vi "PicoScope3000aExampleRapidBlockBulkOverlapped.vi"() -> ()   [LabVIEW 2010]
uses:
  shared/PicoBuffers.ctl
  <vilib>/Waveform/DWDTOps.llb/DWDT Analog to Digital.vi
  shared/Segment Range.ctl
  shared/Buffer and Transfer Settings.ctl
  shared/Acquisition Settings.ctl
  shared/nSegments.ctl
  PicoScope3000aLib/PicoScope3000aDigitalChannelSettings.ctl
  PicoScope3000aLib/PicoScope3000aAnalogChannelSettings.ctl
panel:
  in  "timeIntervalRequested":dbl min=0.0 format="%#6_6p"
  in  "roundFaster":bool=TRUE
  in  "Write to TDMS":bool
  in  "Trigger Settings":T1={"Trigger Enabled"=FALSE, "Trigger Source"=enum."Channel A", "Trigger Threshold (volts)"=0.0, "Trigger Direction"=2, "Trigger Delay (samples)"=0, "Auto Trigger Time (ms)"=1000} {"Trigger Direction" items=["Above", "Below", "Rising", "Falling", "Rising or Falling"]}
  in  "Channel A Settings":T2={"Enabled"=TRUE, "Coupling"=1, "Range"=6, "Analogue Offset"=0.0, "Bandwidth Limit"=0} {"Bandwidth Limit" items=["Full", "20MHz"]; "Range" items=["10 mV", "20 mV", "50 mV", "100 mV", "200 mV", "500 mV", "1 V", "2 V", "5 V", "10 V", "20 V", "50 V ", "100 V"]; "Coupling" items=["AC", "DC"]}
  out "overflow":i16[](array[numeric]) format="%06b"
  in  "Port 0 Settings":T3={"Enabled"=FALSE, "Logic Level"=9830} {"Logic Level" items=["1.5V TTL"=9830, "2.5V CMOS"=16383]}
  out "USB 3.0 device on non-USB 3.0 Port":bool=TRUE
  out "USB Powered":bool=TRUE
  out "Device Info":T4={"Driver Version"="2.1.104.3324", "USB Version"="2.0", "Hardware"="1", "Variant"="5244A", "Batch and Serial"="CQ178/007", "Cal Date"="11Jun13", "Kernel Version"="1.0", "Digital HW Version"="1", "Analogue HW Version"="1", "MSO"=FALSE, "Number of channels"=2}
  in  "Stop Display":bool
  out "Capture Complete":bool
  in  "Run":bool
  in  "Display Buffer Index":i32
  in  "Segment Range":T5={"fromSegmentIndex"=0, "toSegmentIndex"=9} {"toSegmentIndex" format="%.4p"; "fromSegmentIndex" format="%.4p"}
  in  "nSegments":T6=10 format="%.4p"
  out "error out":errorcluster
  in  "Data file":path=path "PicoScope3000aExampleRapidBlock Data"
  in  "Buffer and Transfer Settings":T7={"startIndex"=0, "Samples"=1000000, "Down Sample Ratio"=1, "Down-Sample Mode"=0} {"Down-Sample Mode" items=["RAW none"=2147483648, "None"=0, "Aggregate"=1, "Decimate"=2, "Average"=4]; "Down Sample Ratio" step=1; "Samples" format="%_6p"}
  in  "Acquisition Settings":T8={"preTriggerSamples"=0, "postTriggerSamples"=1000000, "timebase"=5} {"postTriggerSamples" format="%_6p"; "preTriggerSamples" format="%_6p"}
  out "Properties Panel":T9={"Sample Frequency"=41666668.0, "Sample Rate"=2.4000000209412065e-08, "Max Samples Available"=26843008, "Number of Samples"=0, "Total Capture Time (sec) "=0.0, "Max Total Capture Time Available (sec)"=0.6442322134971619} {"Max Total Capture Time Available (sec)" format="%.3p"; "Sample Frequency" format="%.6p"; "Sample Rate" format="%.3p"; "Max Samples Available" format="%_6p"; "Total Capture Time (sec)" format="%.3p"}
  out "Port 0":digitalwaveform(graph)={"t0"=timestamp(0 s since 1904-01-01), "dt"=8e-09, "Y"={"transitions"=[], "data"=[]}}
  in  "stop":bool
  out "Analog Channels":cluster{i32, sgl, "Data":dbl[]}[](graph)
  in  "Serial Number":string
  in  "Use Serial Number":bool
  in  "error in (no error)":errorcluster
  # "Number of\nSegments to Capture"
  # "Bit 0 = ChA"
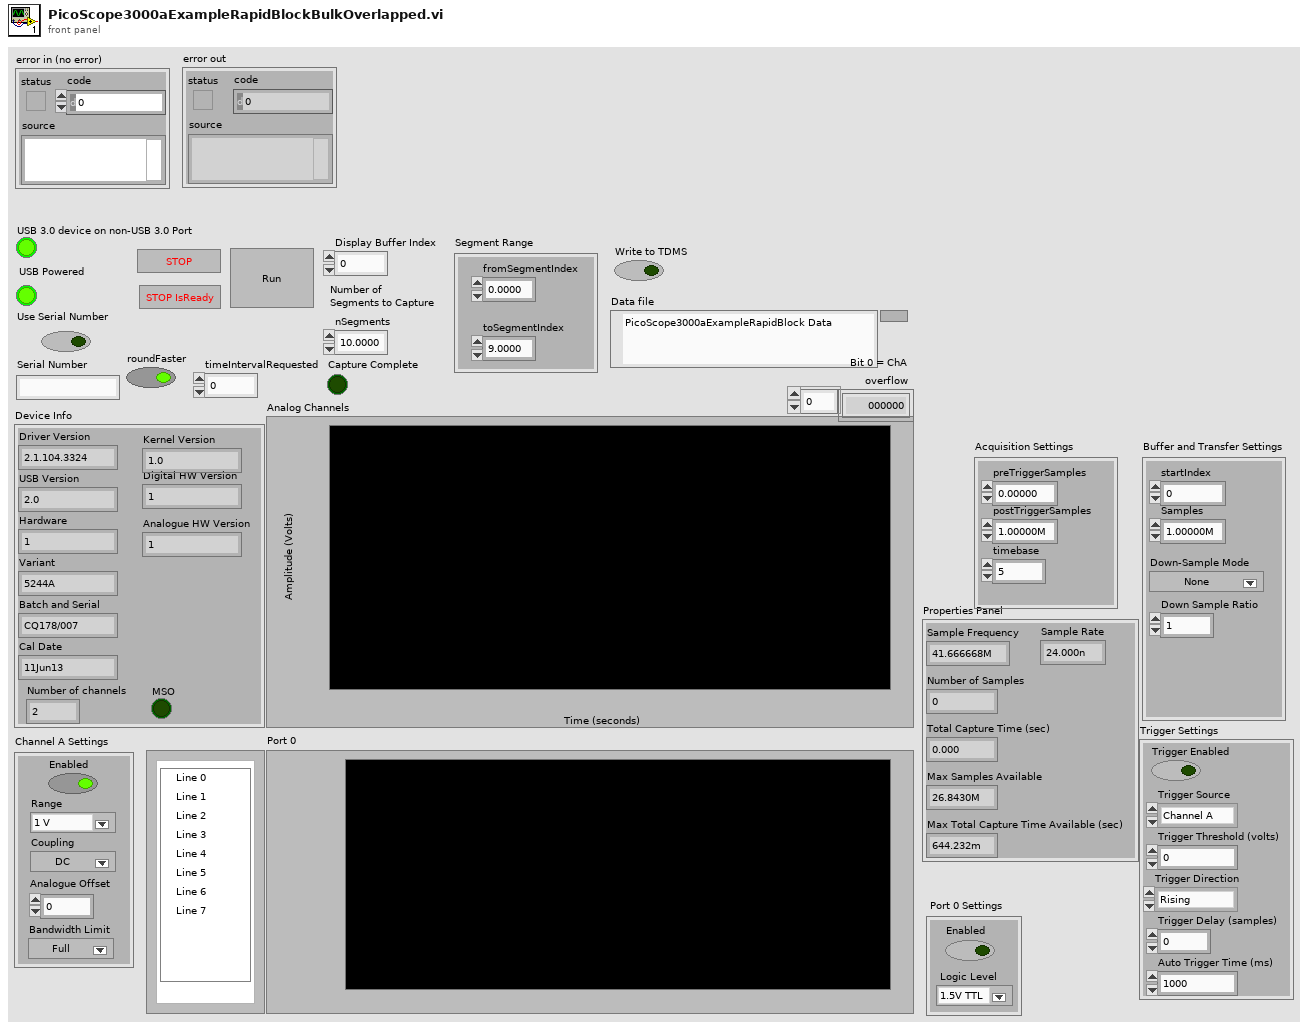
[diagram p1: front panel]
types:
  T1 = cluster{"Trigger Enabled":bool, "Trigger Source":enum32{"Channel A", "Channel B", "Channel C", "Channel D", "Ext."}, "Trigger Threshold (volts)":dbl, "Trigger Direction":u32, "Trigger Delay (samples)":u32, "Auto Trigger Time (ms)":i16}
  T2 = typedef "PicoScope3000aAnalogChannelSettings.ctl" = cluster{"Enabled":bool, "Coupling":u32, "Range":u32, "Analogue Offset":sgl, "Bandwidth Limit":u32}
  T3 = typedef "PicoScope3000aDigitalChannelSettings.ctl" = cluster{"Enabled":bool, "Logic Level":i16}
  T4 = cluster{"Driver Version":string, "USB Version":string, "Hardware":string, "Variant":string, "Batch and Serial":string, "Cal Date":string, "Kernel Version":string, "Digital HW Version":string, "Analogue HW Version":string, "MSO":bool, "Number of channels":i16}
  T5 = typedef "Segment Range.ctl" = cluster{"fromSegmentIndex":u64, "toSegmentIndex":u64}
  T6 = typedef "nSegments.ctl" = u64
  T7 = typedef "Buffer and Transfer Settings.ctl" = cluster{"startIndex":u64, "Samples":u64, "Down Sample Ratio":u64, "Down-Sample Mode":u32}
  T8 = typedef "Acquisition Settings.ctl" = cluster{"preTriggerSamples":u64, "postTriggerSamples":u64, "timebase":u32}
  T9 = cluster{"Sample Frequency":dbl, "Sample Rate":dbl, "Max Samples Available":u64, "Number of Samples":u64, "Total Capture Time (sec) ":dbl, "Max Total Capture Time Available (sec)":dbl}
  T10 = typedef "PicoBuffers.ctl" = cluster{"Max Buffer Pointers":u64[][][], "Min Buffer Pointers":u64[][][], "StreamingDataInfo":cluster{"Channel":u32, "Down-Sample Mode":u32, "PICO_DATA_TYPE":enum32{"PICO_INT8_T", "PICO_INT16_T", "PICO_INT32_T", "PICO_UINT32_T", "PICO_INT64_T", ""}, "Samples":i32, "bufferIndex":u64, "startIndex":i32, "overflow":i16}[][]}
  T11 = enum16{"open", "open or create", "create or replace", "create", "open (read-only)"}
  T12 = cluster{"Sample Frequency":sgl, "Sample Rate":sgl, "Max Samples Available":i32, "Number of Samples":u32, "Total Capture Time (sec) ":sgl, "Max Total Capture Time Available (sec)":sgl}
  T13 = cluster{"Channel A Buffer":i16[], "Channel B Buffer":i16[], "Channel C Buffer":i16[], "Channel D Buffer":i16[], "Channel E Buffer":i16[], "Channel F Buffer":i16[], "Channel G Buffer":i16[], "Channel H Buffer":i16[], "Port 0 Buffer":i16[], "Port 1 Buffer":i16[]}[]
  T14 = cluster{"Channel A Buffer":i16[], "Channel B Buffer":i16[], "Channel C Buffer":i16[], "Channel D Buffer":i16[], "Channel E Buffer":i16[], "Channel F Buffer":i16[], "Channel G Buffer":i16[], "Channel H Buffer":i16[], "Port 0 Buffer":i16[], "Port 1 Buffer":i16[]}
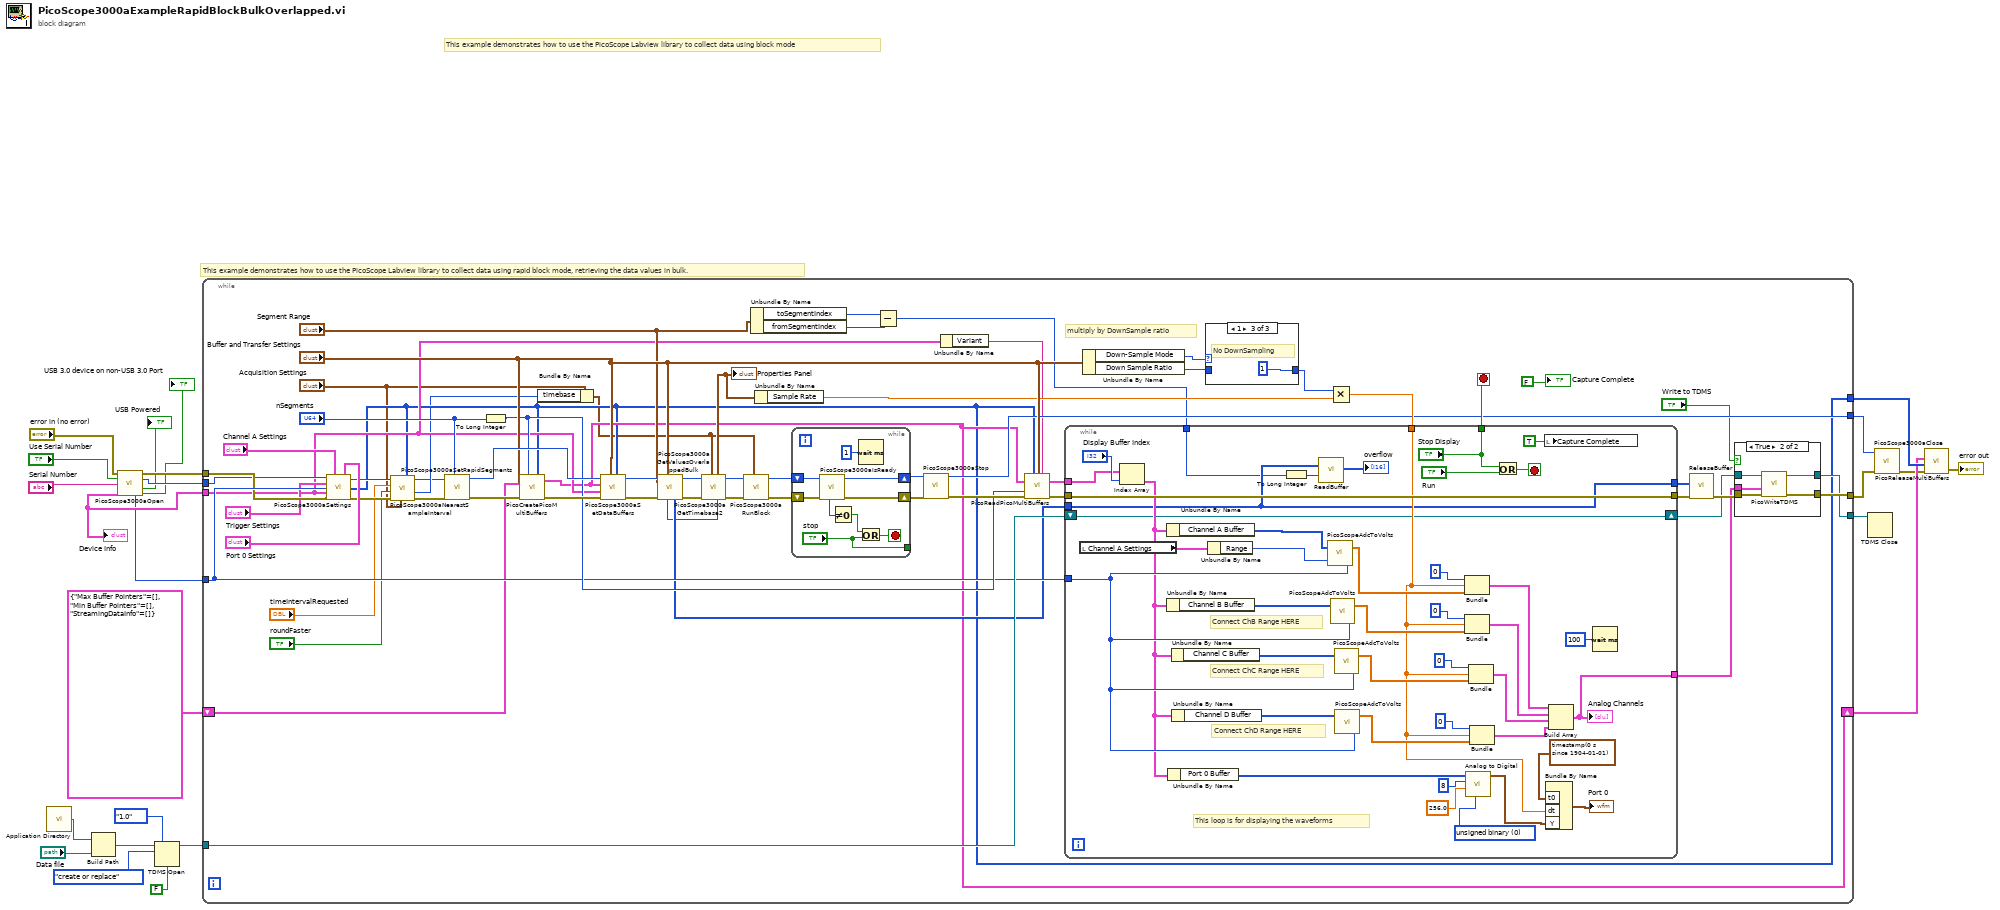
[diagram p0: block diagram]
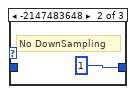
[diagram p4: hidden frame]
diagram:
  # "This example demonstrates how to use the PicoScope Labview library to collect data using rapid block mode, retrieving the data values in bulk."
  # "This example demonstrates how to use the PicoScope Labview library to collect data using block mode"
  n1 = call <vilib>:"Application Directory.vi"() -> ("Application Directory"=w16:path)
  n2 = Build Path(base path=w16, name or relative path="Data file") -> (appended path=w17:path)
  n3 = call "PicoScope3000aOpen.vi"("error in (no error)"="error in (no error)", "Serial Number"="Serial Number", "Use Serial number"="Use Serial Number") -> ("error out"=w8:errorcluster, "handle"=w24:i16, "USB Powered"=→"USB Powered":bool, "Device Info"=w9:T4, "Max ADC value"=w7:i16, "USB 3.0 device on non-USB 3.0 Port"=→"USB 3.0 device on non-USB 3.0 Port":bool)  [unwired: 6 in, 1 out]
  "Device Info" <- w9
  n4 = TDMS Open(6:FALSE ("disable buffering? (T)"), 7:enum16{"1.0", "2.0"}."1.0" ("file format version (2.0)"), 10:T11."create or replace" ("operation (0:open)"), 11:w17) -> (3:w14:refnum<k34>)  [unwired: 2 in, 1 out]
  n5 = while {
    tunnel: w24 -> [w53]
    tunnel: w7 -> [w61]
    tunnel: [w66] -> w22
    tunnel: [w30] -> w23
    tunnel: [w37] -> w15
    tunnel: w14 -> [w86]
    tunnel: w9 -> [w44]
    tunnel: w8 -> [w54]
    tunnel: [w38] -> w2
    shift-right: [w42] -> w3
    shift-left: T10 {"Max Buffer Pointers"=[], "Min Buffer Pointers"=[], "StreamingDataInfo"=[]} ("Data Pointers") -> [w43]
    stop <- w71 stop-if-true
    # "multiply by DownSample ratio"
    n6 = call "PicoScope3000aSettings.vi"("handle in"=w53, "Channel A Settings"="Channel A Settings", "Port 0 Settings"="Port 0 Settings", "Trigger Settings"="Trigger Settings", "Max_adc"=w61, "Device Info"=w44, "error in"=w54) -> ("handle out"=w31:i16, "Enabled Array"=w30:i16[], "error out"=w35:errorcluster)  [unwired: 6 in]
    n7 = call "PicoScope3000aNearestSampleInterval.vi"("Enabled array"=w30, "Acquisition Settings"="Acquisition Settings", "error in (no error)"=w35, "roundFaster"="roundFaster", "timeIntervalRequested"="timeIntervalRequested", "handle in"=w31) -> ("error out"=w34:errorcluster, "timebase"=w27:u32, "handle out"=w26:i16)  [unwired: 2 in, 1 out]
    n8 = call "PicoScope3000aSetRapidSegments.vi"("nSegments"="nSegments", "error in (no error)"=w34, "handle in"=w26) -> ("error out"=w85:errorcluster, "handle out"=w84:i16)  [unwired: 6 in, 1 out]
    n9 = To Long Integer(number="nSegments") -> (32bit integer=w64:i32)
    n10 = call "PicoCreatePicoMultiBuffers.vi"("Number of Buffers"=w64, "Buffer and Transfer Settings"="Buffer and Transfer Settings", "enabled array"=w30, "Data Pointers In"=w43, "error in (no error)"=w85) -> ("Data Pointers"=w42:T10, "error out"=w87:errorcluster)  [unwired: 9 in]
    n11 = Bundle By Name(cluster="Acquisition Settings", "timebase"=w27) -> (w29:T8)
    n12 = call "PicoScope3000aSetDataBuffers.vi"("enabled array"=w30, "Buffer and Transfer Settings"="Buffer and Transfer Settings", "error in (no error)"=w87, "Device Info"=w44, "Data Pointers In"=w42, "handle in"=w84) -> ("error out"=w83:errorcluster, "handle out"=w82:i16)  [unwired: 4 in]
    n13 = call "PicoScope3000aGetValuesOverlappedBulk.vi"("Segment Range"="Segment Range", "Buffer and Transfer Settings"="Buffer and Transfer Settings", "error in (no error)"=w83, "handle in"=w82) -> ("error out"=w58:errorcluster, "handle out"=w57:i16, "Pointer to Overflow"=w50:u64[], "noOfSamples"=w25:u64)  [unwired: 4 in]
    n14 = call "PicoScope3000aGetTimebase2.vi"("Number of Samples"=w25, "Acquisition Settings"=w29, "error in (no error)"=w58, "handle in"=w57) -> ("error out"=w55:errorcluster, "handle out"=w56:i16, "Properties Panel"=w77:T12)  [unwired: 5 in]
    "Properties Panel" <- w77
    n15 = call "PicoScope3000aRunBlock.vi"("Acquisition Settings"=w29, "error in (no error)"=w55, "handle in"=w56) -> ("error out"=w74:errorcluster, "handle out"=w73:i16)  [unwired: 5 in, 2 out]
    n16 = Unbundle By Name("Segment Range") -> ("toSegmentIndex"=w48:u64, "fromSegmentIndex"=w47:u64)
    n17 = Unbundle By Name(w77) -> ("Sample Rate"=w63:sgl)
    n18 = while {
      shift-right: [w144] -> w68
      shift-left: w74 -> [w145]
      shift-right: [w143] -> w65
      shift-left: w73 -> [w142]
      tunnel: ["stop"] -> _
      stop <- w139 stop-if-true
      n19 = call "PicoScope3000aIsReady.vi"("error in (no error)"=w145, "handle in"=w142) -> ("error out"=w144:errorcluster, "handle out"=w143:i16, "ready"=w141:i16)  [unwired: 7 in]
      n20 = Not Equal To 0?(x=w141) -> (x != 0?=w140:bool)
      n21 = Wait (ms)(milliseconds to wait=u32 1) -> ()  [unwired: 1 out]
      n22 = Or(x=w140, y="stop") -> (x .or. y?=w139:bool)
    }
    n23 = Subtract(x=w48, y=w47) -> (x-y=w45:u64)
    n24 = call "PicoScope3000aStop.vi"("error in (no error)"=w68, "handle in"=w65) -> ("error out"=w67:errorcluster, "handle out"=w66:i16)  [unwired: 8 in]
    n25 = Unbundle By Name(w44) -> ("Variant"=w62:string)
    n26 = call "PicoReadPicoMultiBuffers.vi"("enabled array"=w30, "Buffer and Transfer Settings"="Buffer and Transfer Settings", "Variant"=w62, "Data Pointers"=w42, "No of Buffers"=w64, "error in (no error)"=w67) -> ("MultiBuffers (Max or non-aggregated)"=w80:T13, "error out"=w72:errorcluster)  [unwired: 7 in, 1 out]
    n27 = Unbundle By Name("Buffer and Transfer Settings") -> ("Down-Sample Mode"=w78:u32, "Down Sample Ratio"=w79:u64)
    n28 = case shown="1" w78 {
      tunnel: [w146 u64 1 ("Down Sample Ratio") u64 1 ("Down Sample Ratio")] -> w75
      tunnel: w79 -> [w146 _ _]
      frame Default {
      }
      frame -2147483648 {
        # "No DownSampling"
      }
      frame 1 {
        # "No DownSampling"
      }
    }
    n29 = Multiply(x=w75, y=w63) -> (x*y=w76:sgl)
    n30 = while {
      tunnel: w61 -> [w103]
      tunnel: w80 -> [w113]
      tunnel: w76 -> [w105]
      shift-right: [w96] -> w40
      shift-left: w86 -> [w96]
      tunnel: [w119] -> w51
      tunnel: w72 -> [w119]
      tunnel: ["Stop Display"] -> w71
      tunnel: w50 -> [w99]
      tunnel: [w99] -> w49
      tunnel: w45 -> [w98]
      tunnel: [w97] -> w39
      stop <- w116 stop-if-true
      w128 = u16 0 items=["unsigned binary", "offset binary", "2's complement"] ("data format (offset binary)")
      # "This loop is for displaying the waveforms"
      # "Connect ChB Range HERE"
      # "Connect ChD Range HERE"
      # "Connect ChC Range HERE"
      n31 = local read "Channel A Settings"() -> (w95:T2)
      n32 = Index Array(array=w113, index="Display Buffer Index") -> (element=w102:T14)
      n33 = Unbundle By Name(w102) -> ("Channel A Buffer"=w121:i16[])
      n34 = Unbundle By Name(w102) -> ("Channel B Buffer"=w133:i16[])
      n35 = Unbundle By Name(w102) -> ("Port 0 Buffer"=w126:i16[])
      n36 = Unbundle By Name(w102) -> ("Channel C Buffer"=w111:i16[])
      n37 = Unbundle By Name(w102) -> ("Channel D Buffer"=w107:i16[])
      n38 = Unbundle By Name(w95) -> ("Range"=w135:u32)
      n39 = To Long Integer(number=w98) -> (32bit integer=w100:i32)
      n40 = call "ReadBuffer.vi"("Pointer and BufferSize"=w99, "Buffer size"=w100) -> ("Output Array"=→"overflow":i16[])  [unwired: 12 in, 1 out]
      n41 = call "PicoScopeAdcToVolts.vi"("Max_adc"=w103, "Range Index"=w135, "Data"=w121) -> ("Data"=w122:dbl[])
      n42 = call "PicoScopeAdcToVolts.vi"("Max_adc"=w103, "Data"=w133) -> ("Data"=w132:dbl[])  [unwired: 1 in]
      n43 = call "PicoScopeAdcToVolts.vi"("Max_adc"=w103, "Data"=w111) -> ("Data"=w110:dbl[])  [unwired: 1 in]
      n44 = call "PicoScopeAdcToVolts.vi"("Max_adc"=w103, "Data"=w107) -> ("Data"=w106:dbl[])  [unwired: 1 in]
      n45 = Bundle(0, w105, "Data"=w122) -> (w131:cluster{i32, sgl, "Data":dbl[]})  [unwired: 1 in]
      n46 = Bundle(0, w105, "Data"=w132) -> (w130:cluster{i32, sgl, "Data":dbl[]})  [unwired: 1 in]
      n47 = call-poly <vilib>:"Analog to Digital.vi"("data format (offset binary)"=w128, "full-scale range (pk-pk)"=256.0, "resolution (16 bit)"=8, "analog waveform"=w126) -> ("digital waveform"=w123:digitalwaveform)  [unwired: 4 in, 3 out]
      n48 = Bundle(0, w105, "Data"=w110) -> (w109:cluster{i32, sgl, "Data":dbl[]})  [unwired: 1 in]
      n49 = Bundle(0, w105, "Data"=w106) -> (w104:cluster{i32, sgl, "Data":dbl[]})  [unwired: 1 in]
      n50 = Or(x="Stop Display", y="Run") -> (x .or. y?=w116:bool)
      n51 = local write "Capture Complete"(TRUE ("Capture Complete")) -> ()
      n52 = Bundle By Name("t0"=timestamp(0 s since 1904-01-01), "dt"=w105, "Y"=w123) -> (→"Port 0":digitalwaveform)  [unwired: 1 in]
      n53 = Build Array(w131, w130, w109, w104) -> (w97:cluster{i32, sgl, "Data":dbl[]}[])
      "Analog Channels" <- w97
      n54 = Wait (ms)(milliseconds to wait=u32 100) -> ()  [unwired: 1 out]
    }
    n55 = call "ReleaseBuffer.vi"("error in (no error)"=w51, "Pointer and BufferSize"=w49) -> ("error out"=w41:errorcluster)  [unwired: 9 in]
    n56 = case shown="True" "Write to TDMS" {
      tunnel: w39 -> [_ w94]
      tunnel: w40 -> [w88 w93]
      tunnel: w41 -> [w89 w92]
      tunnel: [w89 w91] -> w38
      tunnel: [w88 w90] -> w37
      frame False {
      }
      frame True {
        n57 = call "PicoWriteTDMS.vi"("error in (no error)"=w92, "Analog Channels"=w94, "Refnum in"=w93) -> ("error out"=w91:errorcluster, "Refnum out"=w90:refnum<k34>)  [unwired: 7 in]
      }
    }
    "Capture Complete" <- FALSE ("Capture Complete")
  }
  n58 = TDMS Close(11:w15) -> ()  [unwired: 1 in, 2 out]
  n59 = call "PicoScope3000aClose.vi"("error in (no error)"=w2, "handle in"=w22) -> ("error out"=w1:errorcluster)  [unwired: 8 in, 1 out]
  n60 = call "PicoReleaseMultiBuffers.vi"("error in (no error)"=w1, "Enabled array"=w23, "Data Pointers"=w3) -> ("error out"=→"error out":errorcluster)  [unwired: 7 in, 1 out]
